vi "CV_measure_LCR.vi"(0 "Input parameters":T2={"Measurement type"=enum."Debug", "Sensor type"=enum."HPK_8in_271ch", "Identifier"="test.txt", "Open after execution?"=FALSE, "Plot after execution?"=FALSE, "Display channel"=0, "Voltage Delay (s)"=0.5, "Switch Delay (s)"=0.01, "VISA resource name source"="", "VISA resource name DMM"="", "VISA resource name LCR"="", "Compliance  Level (A)"=10.0, "Voltage Limit (V)"=1000.0, "Data storage location"="", "Scan voltages"="", "Use source as DMM?"=FALSE, "LCR signal frequenzy (Hz)"=10.0, "DMM device"=enum."Keithley2001", "Sampling number"=1, "Use env. sensors on"=enum."Sensirion sht1x/7x", "Switchboard Handle"=0, "Use Switchboard"=FALSE, "LCR signal voltage (V)"=10000.0, "Repeat"=1, "Scan voltages IV"="", "Scan voltages CV"="", "Hex pad numbers?"=FALSE, "Set measurement type"=enum."Debug", "Custom pad scan"="", "IV voltage Delay (s)"=0.5, "CV voltage Delay (s)"=0.5, "Needle measurement?"=FALSE, "Comments"="test.txt", "LCR signal frequenzy (kHz)"=10.0, "Compliance  Level (uA)"=10.0, "Open Correction Array"=array2304x3[6912 elements], "Current set voltage"=0.0, "Last set voltage"=0.0, "Current channel"=0, "Last OpenCorrection index"=-1, "Total curr/vltg every x steps"=10, "Current channel iteration"=0, "No CV corrections"=FALSE, "Mapfile"="", "Corrfile"="", "IV voltage file"=path "", "CV voltage file"=path "", "IV Switch Delay (s)"=0.01, "CV Switch Delay (s)"=0.01, "Invert polarity"=FALSE, "Set debug dirs"=FALSE, "Is n on p"=FALSE, "Source interlock?"=TRUE, "Voltage file used?"=FALSE, "Pad mask"="", "Mask pad above (uA)"=1.0, "LCR device"=enum."LCR_E4980", "Source device"=enum."Source_2410"} {"CV Switch Delay (s)" format="%#_13g"; "IV Switch Delay (s)" format="%#_13g"; "Last set voltage" format="%#_13g"; "Current set voltage" format="%#_13g"; "CV voltage Delay (s)" format="%#_13g"; "IV voltage Delay (s)" format="%#_13g"; "Voltage Limit (V)" format="%#_13g"; "Voltage Delay (s)" format="%#_13g"; "Switch Delay (s)" format="%#_13g"}, 11 "error in (no error)":errorcluster) -> (4 "Input parameters out":T2={"Measurement type"=enum."Debug", "Sensor type"=enum."HPK_8in_271ch", "Identifier"="test.txt", "Open after execution?"=FALSE, "Plot after execution?"=FALSE, "Display channel"=0, "Voltage Delay (s)"=0.5, "Switch Delay (s)"=0.01, "VISA resource name source"="", "VISA resource name DMM"="", "VISA resource name LCR"="", "Compliance  Level (A)"=10.0, "Voltage Limit (V)"=1000.0, "Data storage location"="", "Scan voltages"="", "Use source as DMM?"=FALSE, "LCR signal frequenzy (Hz)"=10.0, "DMM device"=enum."Keithley2001", "Sampling number"=1, "Use env. sensors on"=enum."Sensirion sht1x/7x", "Switchboard Handle"=0, "Use Switchboard"=FALSE, "LCR signal voltage (V)"=10000.0, "Repeat"=1, "Scan voltages IV"="", "Scan voltages CV"="", "Hex pad numbers?"=FALSE, "Set measurement type"=enum."Debug", "Custom pad scan"="", "IV voltage Delay (s)"=0.5, "CV voltage Delay (s)"=0.5, "Needle measurement?"=FALSE, "Comments"="test.txt", "LCR signal frequenzy (kHz)"=10.0, "Compliance  Level (uA)"=10.0, "Open Correction Array"=array2304x3[6912 elements], "Current set voltage"=0.0, "Last set voltage"=0.0, "Current channel"=0, "Last OpenCorrection index"=-1, "Total curr/vltg every x steps"=10, "Current channel iteration"=0, "No CV corrections"=FALSE, "Mapfile"="", "Corrfile"="", "IV voltage file"=path "", "CV voltage file"=path "", "IV Switch Delay (s)"=0.01, "CV Switch Delay (s)"=0.01, "Invert polarity"=FALSE, "Set debug dirs"=FALSE, "Is n on p"=FALSE, "Source interlock?"=TRUE, "Voltage file used?"=FALSE, "Pad mask"="", "Mask pad above (uA)"=1.0, "LCR device"=enum."LCR_E4980", "Source device"=enum."Source_2410"} {"CV Switch Delay (s)" format="%#_13g"; "IV Switch Delay (s)" format="%#_13g"; "Last set voltage" format="%#_13g"; "Current set voltage" format="%#_13g"; "CV voltage Delay (s)" format="%#_13g"; "IV voltage Delay (s)" format="%#_13g"; "Voltage Limit (V)" format="%#_13g"; "Voltage Delay (s)" format="%#_13g"; "Switch Delay (s)" format="%#_13g"}, 8 "LCR data":T1, 15 "error out":errorcluster)   [LabVIEW 2016]
doc: "Measure capacitance and connected quantities from LCR meter."
uses:
  input_params.ctl
  data_LCR.ctl
  <instrlib>/Agilent E4980/Agilent E4980.lvlib
  <instrlib>/Agilent 4263X/Agilent 4263X.lvlib
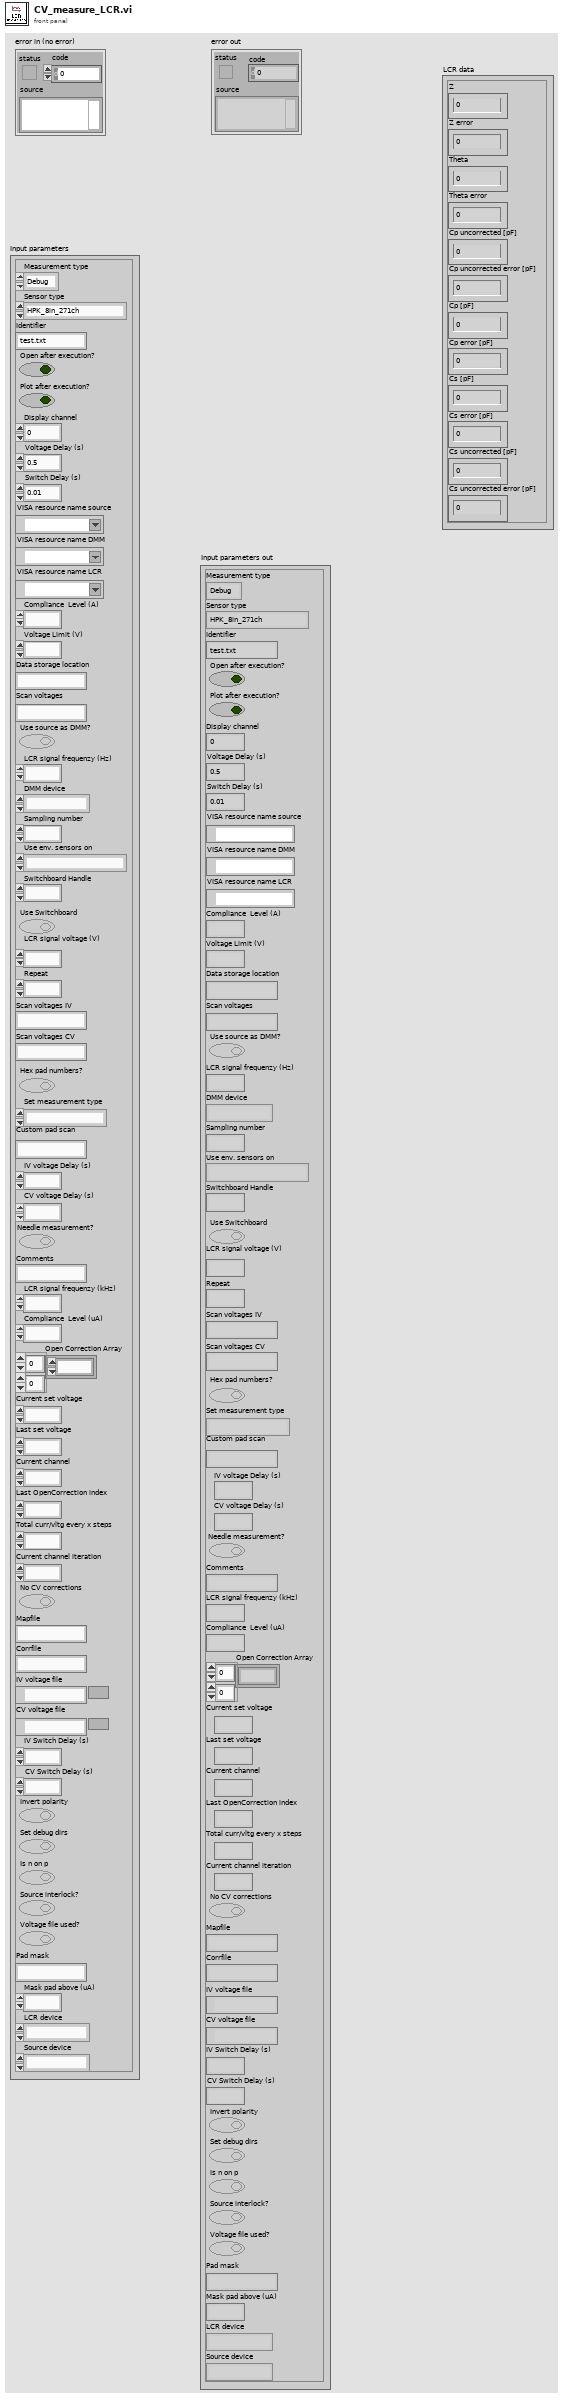
[diagram p1: front panel]
types:
  T1 = typedef "data_LCR.ctl" = cluster{"Z":dbl, "Z error":dbl, "Theta":dbl, "Theta error":dbl, "Cp uncorrected [pF]":dbl, "Cp uncorrected error [pF]":dbl, "Cp [pF]":dbl, "Cp error [pF]":dbl, "Cs [pF]":dbl, "Cs error [pF]":dbl, "Cs uncorrected [pF]":dbl, "Cs uncorrected error [pF]":dbl}
  T2 = typedef "input_params.ctl" = cluster{"Measurement type":enum16{"IV", "CV", "Debug", "Test_contact"}, "Sensor type":enum16{"HPK_6in_135ch", "HPK_8in_271ch", "IFX_8in_256ch", "Diode", "HPK_6in_239ch", "Full_Matrix", "HPK_8in_271ch_full", "HPK_8in_198ch", "LumiCal"}, "Identifier":string, "Open after execution?":bool, "Plot after execution?":bool, "Display channel":i32, "Voltage Delay (s)":dbl, "Switch Delay (s)":dbl, "VISA resource name source":refnum<visa-resource-name>, "VISA resource name DMM":refnum<visa-resource-name>, "VISA resource name LCR":refnum<visa-resource-name>, "Compliance  Level (A)":dbl, "Voltage Limit (V)":dbl, "Data storage location":string, "Scan voltages":string, "Use source as DMM?":bool, "LCR signal frequenzy (Hz)":dbl, "DMM device":enum16{"Keithley2001", "Keithley2450", "Keithley2410", "Keithley6485", "Keithley6487", "Keithley6517"}, "Sampling number":i32, "Use env. sensors on":enum16{"Sensirion sht1x/7x", "Switch Matrix", "Probecard"}, "Switchboard Handle":u32, "Use Switchboard":bool, "LCR signal voltage (V)":dbl, "Repeat":i32, "Scan voltages IV":string, "Scan voltages CV":string, "Hex pad numbers?":bool, "Set measurement type":enum16{"IV", "CV", "Debug", "Test_contact", "IV+CV"}, "Custom pad scan":string, "IV voltage Delay (s)":dbl, "CV voltage Delay (s)":dbl, "Needle measurement?":bool, "Comments":string, "LCR signal frequenzy (kHz)":dbl, "Compliance  Level (uA)":dbl, "Open Correction Array":dbl[][], "Current set voltage":dbl, "Last set voltage":dbl, "Current channel":i32, "Last OpenCorrection index":i32, "Total curr/vltg every x steps":i32, "Current channel iteration":i32, "No CV corrections":bool, "Mapfile":string, "Corrfile":string, "IV voltage file":path, "CV voltage file":path, "IV Switch Delay (s)":dbl, "CV Switch Delay (s)":dbl, "Invert polarity":bool, "Set debug dirs":bool, "Is n on p":bool, "Source interlock?":bool, "Voltage file used?":bool, "Pad mask":string, "Mask pad above (uA)":dbl, "LCR device":enum16{"LCR_E4980", "AGILENT_4263X"}, "Source device":enum16{"Source_2410", "Source_6487"}}
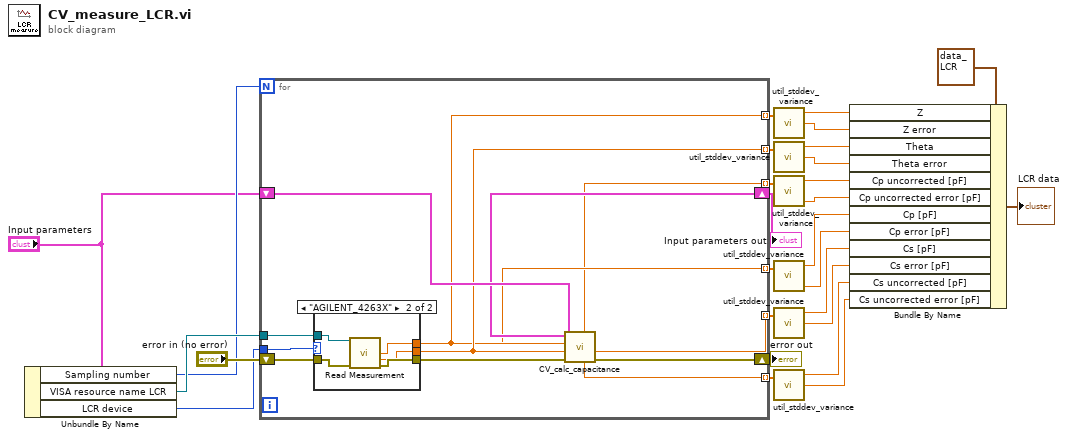
[diagram p0: block diagram]
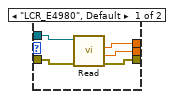
[diagram p2: hidden frame]
diagram:
  n1 = Unbundle By Name("Input parameters") -> ("Sampling number"=w24:i32, "VISA resource name LCR"=w26:refnum<visa-resource-name>, "LCR device"=w1:enum16{"LCR_E4980", "AGILENT_4263X"})
  n2 = for {
    N: w24 -> [_]
    tunnel: w26 -> [w40]
    tunnel: [w32] -> w21 mode=indexing
    tunnel: [w31] -> w20 mode=indexing
    tunnel: [w33] -> w23 mode=indexing
    tunnel: [w34] -> w22 mode=indexing
    shift-right: [w37] -> w27
    shift-left: "error in (no error)" -> [w39]
    tunnel: [w30] -> w17 mode=indexing
    tunnel: [w29] -> w16 mode=indexing
    shift-right: [w35] -> w18
    shift-left: "Input parameters" -> [w36]
    tunnel: w1 -> [w28]
    n3 = case shown="\"AGILENT_4263X\"" w28 {
      tunnel: w40 -> [w45 w50]
      tunnel: w39 -> [w44 w49]
      tunnel: [w41 w48] -> w38
      tunnel: [w42 w46] -> w34
      tunnel: [w43 w47] -> w33
      frame "LCR_E4980", Default {
        n4 = call <instrlib>:"Read.vi"("error in (no error)"=w44, "VISA resource name"=w45) -> ("error out"=w41:errorcluster, "Secondary Parameter"=w42:dbl, "Primary Parameter"=w43:dbl)  [unwired: 6 in, 1 out]
      }
      frame "AGILENT_4263X" {
        n5 = call <instrlib>:"Read Measurement.vi"("VISA resource name"=w50, "error in (no error)"=w49) -> ("primary reading"=w47:dbl, "secondary reading"=w46:dbl, "error out"=w48:errorcluster)  [unwired: 7 in, 4 out]
      }
    }
    n6 = call "CV_calc_capacitance.vi"("error in (no error)"=w38, "Theta (Phase)"=w34, "Z (impedance)"=w33, "Input parameters"=w36) -> ("error out"=w37:errorcluster, "Cs [pF]"=w31:dbl, "Cp [pF]"=w32:dbl, "Input parameters out"=w35:T2, "Cs uncorrected [pF]"=w29:dbl, "Cp uncorrected [pF]"=w30:dbl)  [unwired: 2 in]
  }
  "error out" <- w27
  "Input parameters out" <- w18
  n7 = call "util_stddev_variance.vi"("X"=w23) -> ("mean"=w3:dbl, "standard deviation"=w4:dbl)  [unwired: 1 in, 1 out]
  n8 = call "util_stddev_variance.vi"("X"=w22) -> ("mean"=w2:dbl, "standard deviation"=w5:dbl)  [unwired: 1 in, 1 out]
  n9 = call "util_stddev_variance.vi"("X"=w17) -> ("mean"=w6:dbl, "variance"=w7:dbl)  [unwired: 1 in, 1 out]
  n10 = call "util_stddev_variance.vi"("X"=w21) -> ("mean"=w8:dbl, "variance"=w9:dbl)  [unwired: 1 in, 1 out]
  n11 = call "util_stddev_variance.vi"("X"=w20) -> ("mean"=w10:dbl, "standard deviation"=w11:dbl)  [unwired: 1 in, 1 out]
  n12 = call "util_stddev_variance.vi"("X"=w16) -> ("mean"=w12:dbl, "standard deviation"=w13:dbl)  [unwired: 1 in, 1 out]
  n13 = Bundle By Name(cluster=T1 {"Z"=0.0, "Z error"=0.0, "Theta"=0.0, "Theta error"=0.0, "Cp uncorrected [pF]"=0.0, "Cp uncorrected error [pF]"=0.0, "Cp [pF]"=0.0, "Cp error [pF]"=0.0, "Cs [pF]"=0.0, "Cs error [pF]"=0.0, "Cs uncorrected [pF]"=0.0, "Cs uncorrected error [pF]"=0.0} ("Cluster"), "Z"=w3, "Z error"=w4, "Theta"=w2, "Theta error"=w5, "Cp uncorrected [pF]"=w6, "Cp uncorrected error [pF]"=w7, "Cp [pF]"=w8, "Cp error [pF]"=w9, "Cs [pF]"=w10, "Cs error [pF]"=w11, "Cs uncorrected [pF]"=w12, "Cs uncorrected error [pF]"=w13) -> (→"LCR data":T1)
